vi "indices.vi"(4 "corriente laser":i32, 5 "voltaje":i32, 6 "polarizador":i32, 7 "espejo":i32, 8 "indice 3":i32, 9 "indice 2":i32, 10 "indice 1":i32, 11 "Orden":T1(array[ring])=[enum."espejos", enum."voltaje", enum."polarizador", enum."potenciometro ", enum."CCD"]) -> (1 "INDICES 2":i32[](array[numeric]), 2 "dimensiones":i32[](array[numeric]))   [LabVIEW 2016]
panel:
  out "Array":i32[](array[numeric])
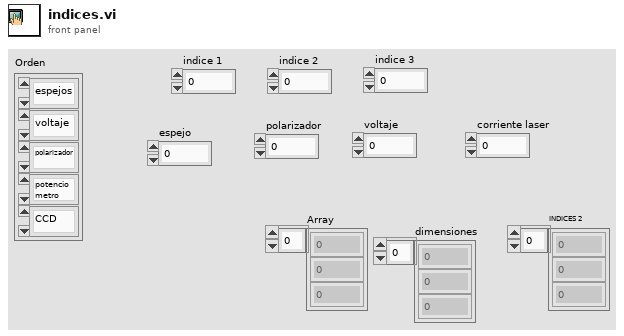
[diagram p1: front panel]
types:
  T1 = enum16{"espejos", "polarizador", "voltaje", "potenciometro ", "CCD", "lockin", "laser", "ninguno"}[]
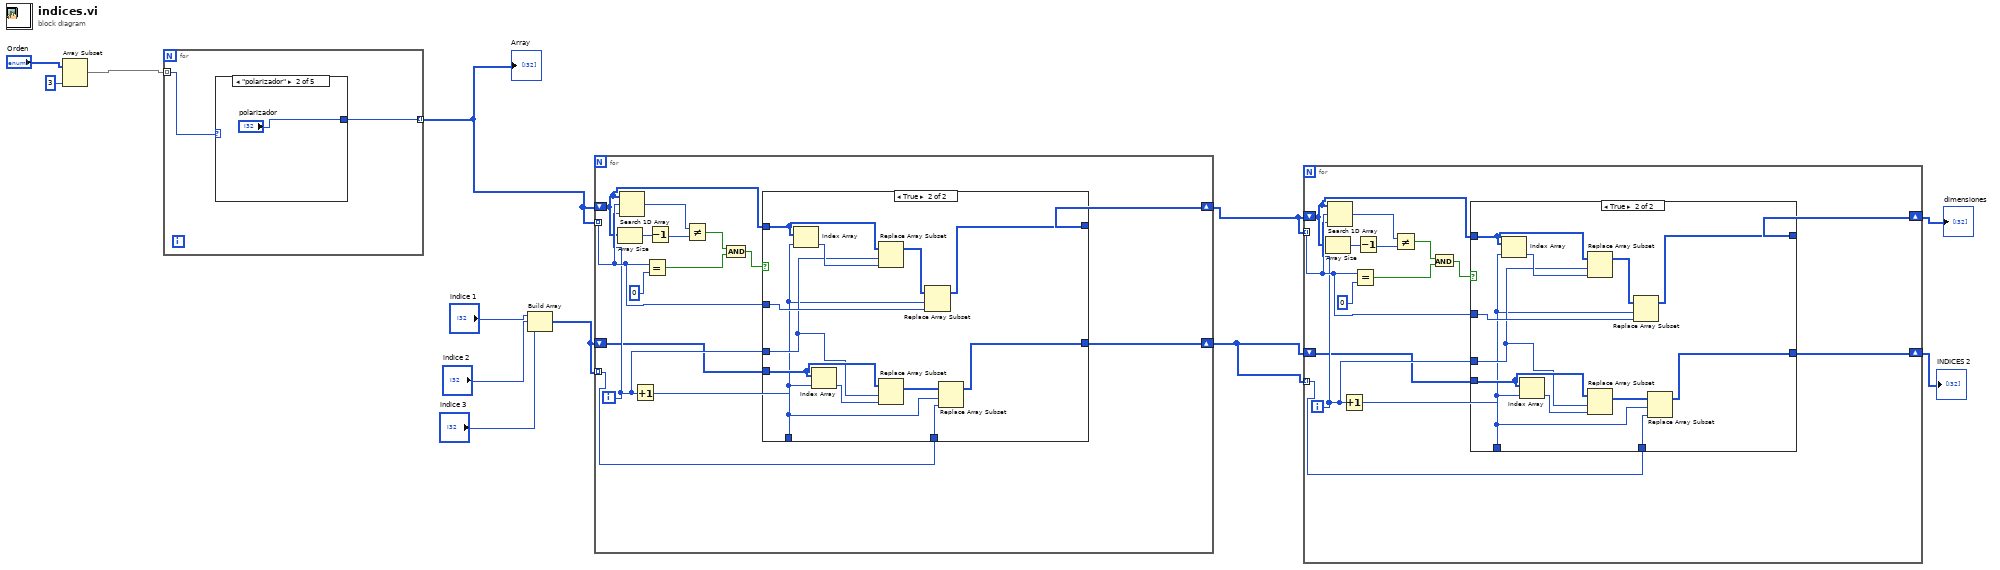
[diagram p0: block diagram]
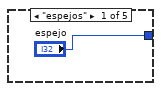
[diagram p4: hidden frame]
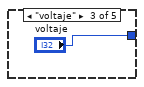
[diagram p5: hidden frame]
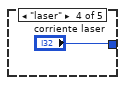
[diagram p6: hidden frame]
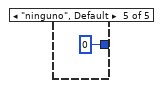
[diagram p7: hidden frame]
diagram:
  n1 = Array Subset(array="Orden", length=3) -> (w10:T1)  [unwired: 1 in]
  n2 = for {
    tunnel: w10 -> [w14] mode=indexing
    tunnel: [w13] -> w9 mode=indexing
    n3 = case shown="\"polarizador\"" w14 {
      tunnel: ["espejo" "polarizador" "voltaje" "corriente laser" 0 ("corriente laser")] -> w13
      frame "espejos" {
      }
      frame "polarizador" {
      }
      frame "voltaje" {
      }
      frame "laser" {
      }
      frame "ninguno", Default {
      }
    }
  }
  "Array" <- w9
  n4 = Build Array("indice 1", "indice 2", "indice 3") -> (w5:i32[])
  n5 = for {
    tunnel: w9 -> [w26] mode=indexing
    shift-right: [w24] -> w2
    shift-left: w9 -> [w23]
    shift-right: [w20] -> w1
    shift-left: w5 -> [w22]
    tunnel: w5 -> [w21] mode=indexing
    i -> [w25]
    n6 = Array Size(array=w23) -> (size(s)=w33:i32)
    n7 = Search 1D Array(1D array=w23, element=w26, start index (0)=w25) -> (index of element=w31:i32)
    n8 = Increment(x=w25) -> (x+1=w27:i32)
    n9 = Equal?(x=w26, y=0) -> (x = y?=w29:bool)
    n10 = Decrement(x=w33) -> (x-1=w32:i32)
    n11 = Not Equal?(x=w31, y=w32) -> (x != y?=w30:bool)
    n12 = And(x=w30, y=w29) -> (x .and. y?=w28:bool)
    n13 = case shown="True" w28 {
      tunnel: w23 -> [w36 w46]
      tunnel: w27 -> [_ w39]
      tunnel: w26 -> [_ w47]
      tunnel: w25 -> [_ w42]
      tunnel: [w36 w44] -> w24
      tunnel: w22 -> [w35 w43]
      tunnel: w21 -> [_ w38]
      tunnel: [w35 w37] -> w20
      frame False {
      }
      frame True {
        n14 = Index Array(array=w46, index=w39) -> (element=w48:i32)
        n15 = Index Array(array=w43, index=w39) -> (element=w41:i32)
        n16 = Replace Array Subset(array=w46, new element=w48, index=w42) -> (w45:i32[])
        n17 = Replace Array Subset(array=w43, new element=w41, index=w42) -> (w40:i32[])
        n18 = Replace Array Subset(array=w45, new element=w47, index=w39) -> (w44:i32[])
        n19 = Replace Array Subset(array=w40, new element=w38, index=w39) -> (w37:i32[])
      }
    }
  }
  n20 = for {
    tunnel: w2 -> [w55] mode=indexing
    shift-right: [w53] -> w4
    shift-left: w2 -> [w52]
    shift-right: [w49] -> w3
    shift-left: w1 -> [w51]
    tunnel: w1 -> [w50] mode=indexing
    i -> [w54]
    n21 = Array Size(array=w52) -> (size(s)=w62:i32)
    n22 = Search 1D Array(1D array=w52, element=w55, start index (0)=w54) -> (index of element=w60:i32)
    n23 = Increment(x=w54) -> (x+1=w56:i32)
    n24 = Equal?(x=w55, y=0) -> (x = y?=w58:bool)
    n25 = Decrement(x=w62) -> (x-1=w61:i32)
    n26 = Not Equal?(x=w60, y=w61) -> (x != y?=w59:bool)
    n27 = And(x=w59, y=w58) -> (x .and. y?=w57:bool)
    n28 = case shown="True" w57 {
      tunnel: w52 -> [w65 w75]
      tunnel: w56 -> [_ w68]
      tunnel: w55 -> [_ w76]
      tunnel: w54 -> [_ w71]
      tunnel: [w65 w73] -> w53
      tunnel: w51 -> [w64 w72]
      tunnel: w50 -> [_ w67]
      tunnel: [w64 w66] -> w49
      frame False {
      }
      frame True {
        n29 = Index Array(array=w75, index=w68) -> (element=w77:i32)
        n30 = Index Array(array=w72, index=w68) -> (element=w70:i32)
        n31 = Replace Array Subset(array=w75, new element=w77, index=w71) -> (w74:i32[])
        n32 = Replace Array Subset(array=w72, new element=w70, index=w71) -> (w69:i32[])
        n33 = Replace Array Subset(array=w74, new element=w76, index=w68) -> (w73:i32[])
        n34 = Replace Array Subset(array=w69, new element=w67, index=w68) -> (w66:i32[])
      }
    }
  }
  "dimensiones" <- w4
  "INDICES 2" <- w3
